vi "Move_org.vi"(0 "X":dbl, 1 "Absolute":bool=TRUE, 5 "Y":dbl, 7 "Z":dbl, 9 "SpeedXY (mm/s)":dbl=100.0, 11 "SpeedZ (mm/s)":dbl=10.0, 12 "Move Z first":bool) -> (4 "Position Gcode":string, 15 "error out":errorcluster)   [LabVIEW 2019]
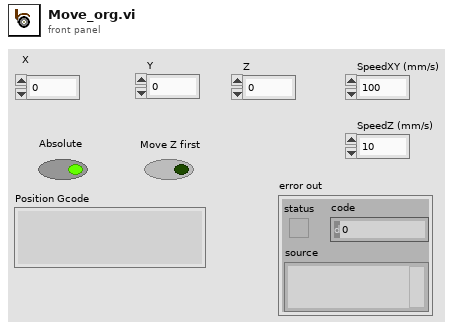
[diagram p1: front panel]
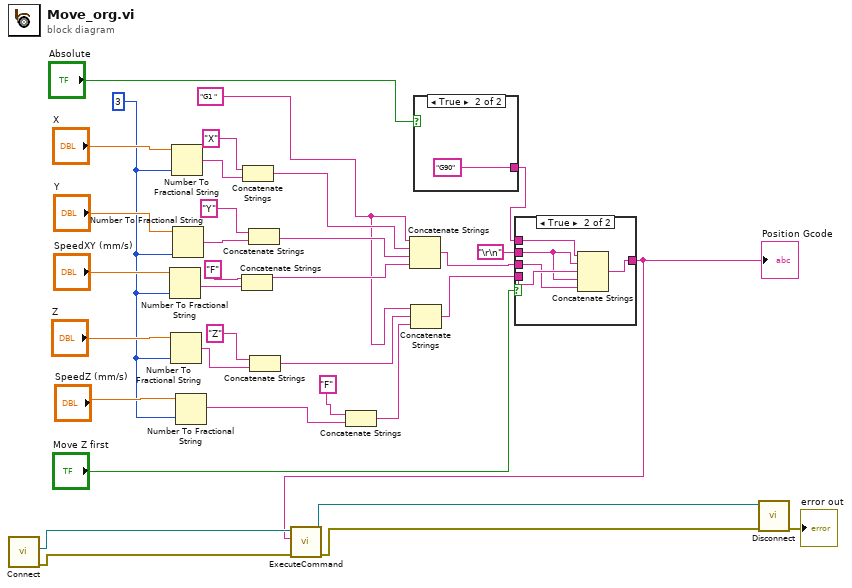
[diagram p0: block diagram]
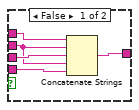
[diagram p2: hidden frame]
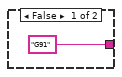
[diagram p3: hidden frame]
diagram:
  w14 = "G1 " ("string")
  w17 = 3
  n1 = call "Connect.vi"() -> ("error out"=w5:errorcluster, "controller"=w6:refnum<k24>)  [unwired: 10 in]
  n2 = Number To Fractional String(number="SpeedXY (mm/s)", precision (6)=w17) -> (F-format string=w22:string)  [unwired: 2 in]
  n3 = Number To Fractional String(number="Z", precision (6)=w17) -> (F-format string=w25:string)  [unwired: 2 in]
  n4 = Number To Fractional String(number="X", precision (6)=w17) -> (F-format string=w32:string)  [unwired: 2 in]
  n5 = Number To Fractional String(number="Y", precision (6)=w17) -> (F-format string=w30:string)  [unwired: 2 in]
  n6 = Number To Fractional String(number="SpeedZ (mm/s)", precision (6)=w17) -> (F-format string=w16:string)  [unwired: 2 in]
  n7 = Concatenate Strings("F", w22) -> (w20:string)
  n8 = Concatenate Strings("X", w32) -> (w28:string)
  n9 = Concatenate Strings("Y", w30) -> (w27:string)
  n10 = Concatenate Strings("Z", w25) -> (w13:string)
  n11 = Concatenate Strings("F", w16) -> (w12:string)
  n12 = Concatenate Strings(w14, w28, w27, w20) -> (w9:string)
  n13 = Concatenate Strings(w14, w13, w12) -> (w8:string)
  n14 = case shown="True" "Absolute" {
    tunnel: ["G91" "G90"] -> w11
    frame False {
    }
    frame True {
    }
  }
  n15 = case shown="True" "Move Z first" {
    tunnel: w11 -> [w41 w45]
    tunnel: "\r\n" -> [w39 w43]
    tunnel: w9 -> [w40 w42]
    tunnel: w8 -> [w38 w44]
    tunnel: [w37 w46] -> w4
    frame False {
      n16 = Concatenate Strings(w41, w39, w40, w39, w38) -> (w37:string)
    }
    frame True {
      n17 = Concatenate Strings(w45, w43, w44, w43, w42) -> (w46:string)
    }
  }
  "Position Gcode" <- w4
  n18 = call "ExecuteCommand.vi"("error in (no error)"=w5, "Command Code"=w4, "controller in"=w6) -> ("error out"=w2:errorcluster, "controller out"=w3:refnum<k24>)  [unwired: 6 in, 1 out]
  n19 = call "Disconnect.vi"("error in (no error)"=w2, "controller"=w3) -> ("error out"=→"error out":errorcluster)  [unwired: 9 in]
